vi "GenerateEventItemBuilt.vi"(9 "ProjectItem":refnum<class "ProjectItem.lvclass">, 10 "Result":string, 11 "ItemBuilt":T1) -> ()   [LabVIEW 2019, in "SolutionBuilder.lvlib" / "ProjectItem.lvclass"]
uses:
  ProjectItem.lvclass
  Events/EventItemBuilt.ctl
  SolutionBuilder.lvlib
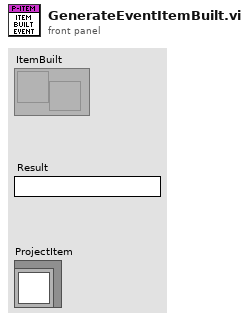
[diagram p1: front panel]
types:
  T1 = typedef "SolutionBuilder.lvlib/EventItemBuilt.ctl" = refnum<user-event>
  T2 = cluster{"Build spec name":string, "Target":string, "name":string, "Result":string}
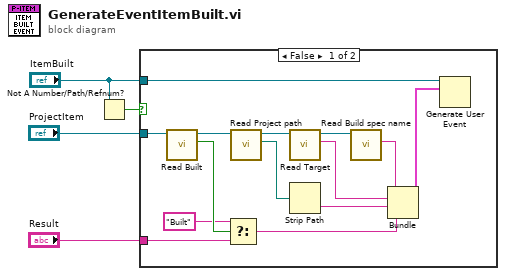
[diagram p0: block diagram]
diagram:
  n1 = Not A Number/Path/Refnum?(number/path/refnum="ItemBuilt") -> (NaN/Path/Refnum?=w1:bool)
  n2 = case shown="False" w1 {
    tunnel: "ProjectItem" -> [w18 _]
    tunnel: "Result" -> [w9 _]
    tunnel: "ItemBuilt" -> [w8 _]
    frame False {
      n3 = call-dynamic "Read Built.vi"("ProjectItem in"=w18) -> ("Built"=w13:bool, "ProjectItem out"=w17:refnum<class "ProjectItem.lvclass">)  [unwired: 9 in]
      n4 = Select(t="Built" ("name"), s=w13, f=w9) -> (s? t:f=w11:string)
      n5 = call-dynamic "Read Project path.vi"("ProjectItem in"=w17) -> ("Project path"=w15:path, "ProjectItem out"=w7:refnum<class "ProjectItem.lvclass">)  [unwired: 9 in]
      n6 = call "Read Target.vi"("ProjectItem in"=w7) -> ("Target"=w5:string, "ProjectItem out"=w6:refnum<class "ProjectItem.lvclass">)  [unwired: 9 in]
      n7 = Strip Path(path=w15) -> (name=w14:string)  [unwired: 1 out]
      n8 = call-dynamic "Read Build spec name.vi"("ProjectItem in"=w6) -> ("Build spec name"=w16:string)  [unwired: 9 in, 1 out]
      n9 = Bundle("Build spec name"=w16, "Target"=w5, "name"=w14, "Result"=w11) -> (w10:T2)  [unwired: 1 in]
      n10 = Generate User Event(user event=w8, event data cluster=w10) -> ()  [unwired: 2 in, 2 out]
    }
    frame True {
    }
  }
